vi "Init Port.vi"(8 "error in (no error)":errorcluster, 10 "BAUD":u16, 11 "String":string) -> (0 "error out":errorcluster, 3 "VISA Refnum out":refnum<visa-resource-name>)   [LabVIEW 2020]
uses:
  <vilib>/Instr/_visa.llb/VISA Open Access Mode.ctl
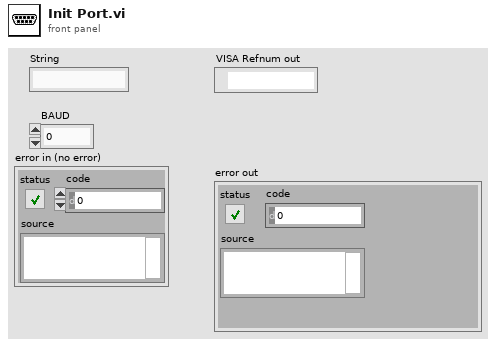
[diagram p1: front panel]
types:
  T1 = typedef "VISA Open Access Mode.ctl" = u32
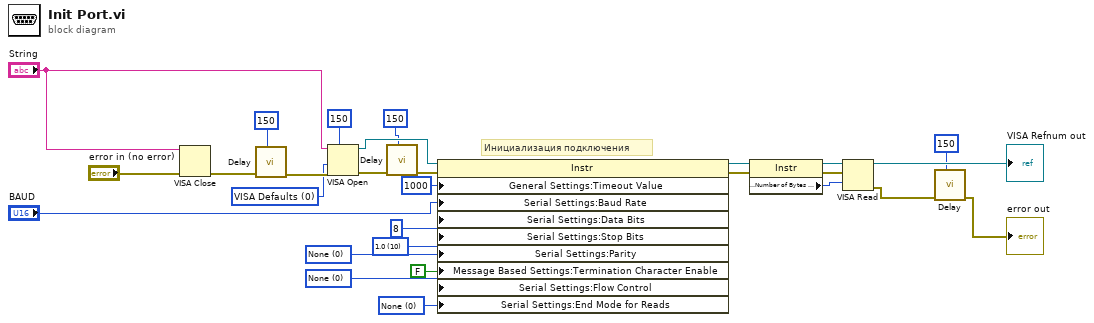
[diagram p0: block diagram]
diagram:
  w2 = T1 0 items=["VISA Defaults"=0, "Exclusive Lock"=1, "Load Configured Settings"=4] ("Access Mode")
  w28 = u16 0 items=["None", "Odd", "Even", "Mark", "Space"] ("Serial Settings:Parity")
  w26 = u16 0 items=["None", "XON/XOFF", "RTS/CTS", "XON/XOFF & RTS/CTS", "DTR/DSR", "XON/XOFF & DTR/DSR"] ("Serial Settings:Flow Control")
  w13 = u16 0 items=["None", "LastBit", "TermChar"] ("Serial Settings:Serial End Mode for Reads")
  w11 = u16 10 items=["1.0"=10, "1.5"=15, "2.0"=20] ("Serial Settings:Serial Stop Bits")
  # "Инициализация подключения"
  n1 = VISA Close(VISA resource name="String", error in (no error)="error in (no error)") -> (error out=w6:errorcluster)
  n2 = call "Delay.vi"("milliseconds to wait"=u32 150, "error in (no error)"=w6) -> ("error out"=w5:errorcluster)  [unwired: 8 in, 1 out]
  n3 = VISA Open(timeout (0)=u32 150 ("VISA Open timeout (0)"), access mode=w2, error in (no error)=w5, VISA resource name="String") -> (VISA resource name=w21:refnum<visa-resource-name>, error out=w18:errorcluster)  [unwired: 1 in]
  n4 = call "Delay.vi"("milliseconds to wait"=u32 150, "error in (no error)"=w18) -> ("error out"=w19:errorcluster)  [unwired: 8 in, 1 out]
  n5 = property class="Instr"(reference=w21, error in=w19, "General Settings:Timeout Value"=u32 1000, "Serial Settings:Baud Rate"="BAUD", "Serial Settings:Data Bits"=u16 8 ("data bits"), "Serial Settings:Stop Bits"=w11, "Serial Settings:Parity"=w28, "Message Based Settings:Termination Character Enable"=FALSE, "Serial Settings:Flow Control"=w26, "Serial Settings:End Mode for Reads"=w13) -> (reference out=w15:refnum<visa-resource-name>, error out=w25:errorcluster)
  n6 = property class="Instr"(reference=w15, error in=w25) -> (reference out=w22:refnum<visa-resource-name>, error out=w20:errorcluster, "Serial Settings:Number of Bytes at Serial Port"=w17:u32)
  n7 = VISA Read(VISA resource name=w22, byte count=w17, error in (no error)=w20) -> (VISA resource name out=→"VISA Refnum out":refnum<visa-resource-name>, error out=w10:errorcluster)  [unwired: 2 out]
  n8 = call "Delay.vi"("milliseconds to wait"=u32 150, "error in (no error)"=w10) -> ("error out"=→"error out":errorcluster)  [unwired: 8 in, 1 out]
